vi "Get Scalar Data Variant.vi"(8 "error in (no error)":errorcluster, 9 "index":i32, 11 "Core Transfers Configuration in":refnum<class "Core Transfers Configuration.lvclass">) -> (0 "error out":errorcluster, 1 "data version":T1, 2 "data":variant, 3 "Core Transfers Configuration out":refnum<class "Core Transfers Configuration.lvclass">)   [LabVIEW 2017, in "DSF Core.lvlib" / "Core Transfers Configuration.lvclass"]
uses:
  Core Transfers Configuration.lvclass
  C:/Git/DSF/Core/Classes/Configuration/Configuration.lvclass
  Typedefs/DSF Version Info.ctl
  Configuration.lvclass
  DSF Core.lvlib
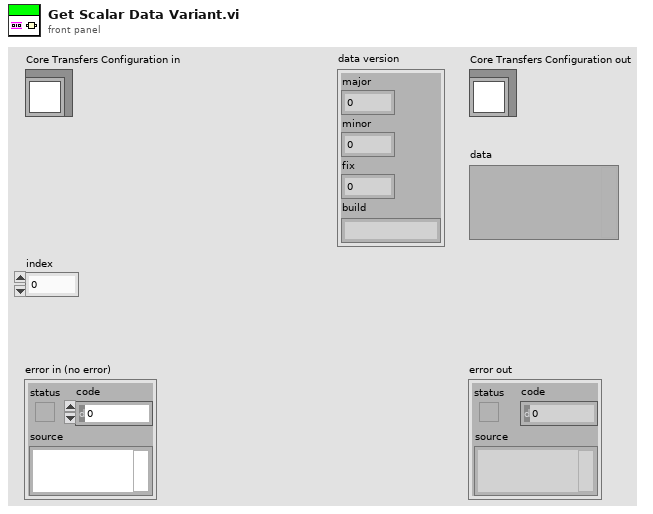
[diagram p1: front panel]
types:
  T1 = typedef "DSF Core.lvlib/DSF Version Info.ctl" = cluster{"major":i32, "minor":i32, "fix":i32, "build":string}
  T2 = typedef "DSF Core.lvlib/Core Transfers Configuration.lvclass/Configuration.ctl" = cluster{"name":string}
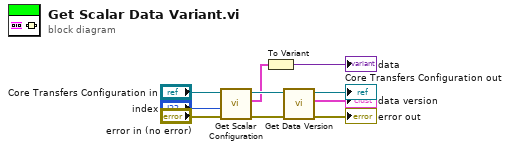
[diagram p0: block diagram]
diagram:
  n1 = call "Get Scalar Configuration.vi"("error in (no error)"="error in (no error)", "index"="index", "Core Transfers Configuration in"="Core Transfers Configuration in") -> ("error out"=w6:errorcluster, "transfer configuration"=w4:T2, "Core Transfers Configuration out"=w5:refnum<class "Core Transfers Configuration.lvclass">)  [unwired: 6 in]
  n2 = To Variant(anything=w4) -> (Variant=→"data":variant)
  n3 = call "Get Data Version.vi"("error in (no error)"=w6, "Configuration in"=w5) -> ("error out"=→"error out":errorcluster, "data version"=→"data version":T1, "Configuration out"=→"Core Transfers Configuration out":refnum<class "Core Transfers Configuration.lvclass">)  [unwired: 7 in]
